vi "FTW-TransferClient-DownloadBegin.vi"(0 "Transfer Client":refnum<class "FTW-TransferClient.lvclass">, 5 "Local Filepath":path, 7 "Remote Relative Filepath":string, 11 "error in":errorcluster) -> (4 "Transfer Client out":refnum<class "FTW-TransferClient.lvclass">, 6 "Download Events":refnum<event-registration>, 15 "error out":errorcluster)   [LabVIEW 2014, in "FTW-TransferClient.lvclass"]
uses:
  FTW-TransferClient.lvclass
  FTW-TransferClient-TransferProgress.ctl
  FTW-TransferClient-TransferStatus.ctl
  core/error/FTW-ERR-Assert-DeveloperError.vi
  core/error/FTW-ERR-ThrowError.vi
  core/error/FTW-ERR-NoErrorConstant.vi
  core/error/FTW-ERR-CallChain.vi
  core/string/FTW-STR-ReplaceWhitespace.vi
panel:
  # "Inputs"
  # "Outputs"
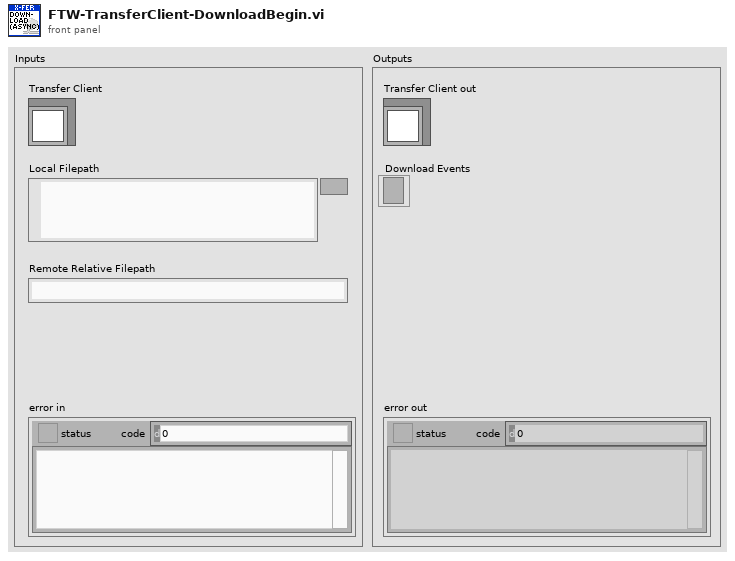
[diagram p1: front panel]
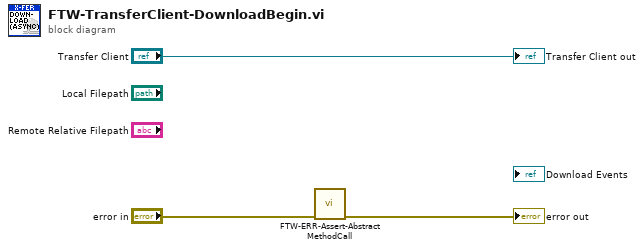
[diagram p0: block diagram]
diagram:
  n1 = call "FTW-ERR-Assert-AbstractMethodCall.vi"("error in"="error in") -> ("error out"=→"error out":errorcluster)  [unwired: 14 in]
  "Transfer Client out" <- "Transfer Client"
